vi "OKNrunge4th.vi"(8 "Integration time":dbl=0.01 format="%#_13g", 9 "r_slip":dbl, 10 "Storage K":dbl, 11 "f(0)":dbl format="%#_13g") -> (3 "f'(x)":dbl)   [LabVIEW 2016]
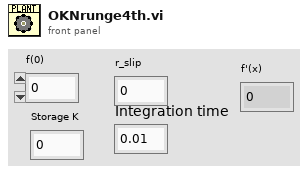
[diagram p1: front panel]
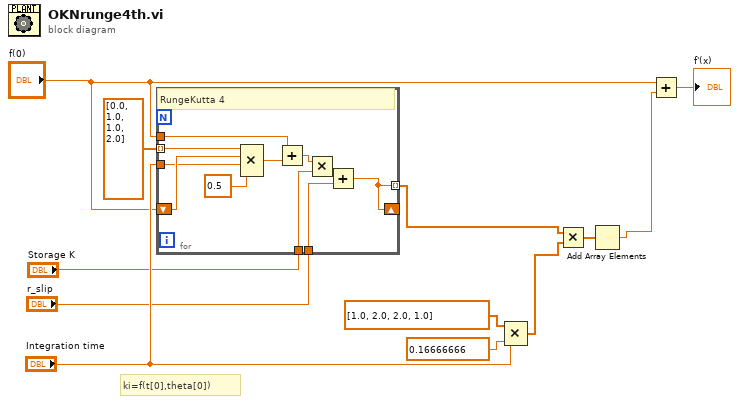
[diagram p0: block diagram]
diagram:
  # "ki=f(t[0],theta[0])"
  n1 = for {
    shift-right: [w13] -> _
    shift-left: "f(0)" -> [w23]
    tunnel: "f(0)" -> [w21]
    tunnel: dbl[] [0.0, 1.0, 1.0, 2.0] ("k") -> [w20] mode=indexing
    tunnel: "Integration time" -> [w18]
    tunnel: "Storage K" -> [w16]
    tunnel: "r_slip" -> [w14]
    tunnel: [w13] -> w5 mode=indexing
    # "RungeKutta 4"
    n2 = Compound Arithmetic op=MULTIPLY(w20, w23, w18, 0.5 ("value")) -> (w22:dbl)
    n3 = Add(x=w21, y=w22) -> (x+y=w17:dbl)
    n4 = Multiply(x=w17, y=w16) -> (x*y=w15:dbl)
    n5 = Add(x=w15, y=w14) -> (x+y=w13:dbl)
  }
  n6 = Compound Arithmetic op=MULTIPLY(dbl[] [1.0, 2.0, 2.0, 1.0] ("k"), "Integration time", 0.16666666 ("value")) -> (w4:dbl[])
  n7 = Multiply(x=w5, y=w4) -> (x*y=w3:dbl[])
  n8 = Add Array Elements(numeric array=w3) -> (sum=w2:dbl)
  n9 = Add(x="f(0)", y=w2) -> (x+y=→"f'(x)":dbl)
